vi "SwerveDriveSwerveWheel.vi"(0 "Wheel_Encoder":T1={"DevStatus"={"status"=FALSE, "code"=0, "source"=""}, "Analog Channel"=enum."Invalid"}, 1 "Wheel_Position":string="Numeric Array", 2 "Inputs":dbl[](array[numeric]), 3 "Length":dbl, 4 "Center":dbl, 5 "error in (no error)":errorcluster, 6 "Wheel_Offset":dbl, 7 "Width":dbl, 8 "MotorControlDevRef":T3={"DeviceStatus"={"status"=FALSE, "code"=0, "source"=""}, "Type"=enum."PWM", "PWM"={"PWM Channel"=enum."Invalid", "DeadBand"={"Name"="", "maxPositivePwm"=0, "minPositivePwm"=0, "centerPwm"=0, "maxNegativePwm"=0, "minNegativePwm"=0, "angularRange"=0}}, "CAN"={"Device Number"=0, "SetOutput VI Ref"=variant(refnum<vi> refnum), "GetOutput VI Ref"=variant(refnum<vi> refnum), "Enable VI Ref"=variant(refnum<vi> refnum), "Disable VI Ref"=variant(refnum<vi> refnum), "Data"=variant}, "Invert"=FALSE, "DIO PWM"={"PWM \"Enable\" Channel"=enum."Invalid", "DIOChannel"=enum."Invalid", "PWM Rate"=0.0}}) -> (19 "Speed":dbl)   [LabVIEW 2019, in "Swerve Drive.lvlib"]
uses:
  Swerve Drive.lvlib
  <vilib>/Rock Robotics/WPI/MotorControl/WPI_MotorControlDeviceRef.ctl
  <vilib>/Rock Robotics/WPI/MotorControl/WPI_MotorControlType.ctl
  <vilib>/Rock Robotics/SystemInterfaces/DIO/FPGA_DIOPWMChannel.ctl
  <vilib>/Rock Robotics/WPI/PWM/WPI_PWMDeadband.ctl
  <vilib>/Rock Robotics/SystemInterfaces/DIO/FPGA_DIOChannel.ctl
  <vilib>/Rock Robotics/WPI/AnalogChannel/WPI_AnalogChannelDevRef.ctl
  <vilib>/Rock Robotics/SystemInterfaces/AI/FPGA_AIChannel.ctl
  <vilib>/Rock Robotics/Network Tables/NT Write Number.vi
panel:
  out "error out":errorcluster
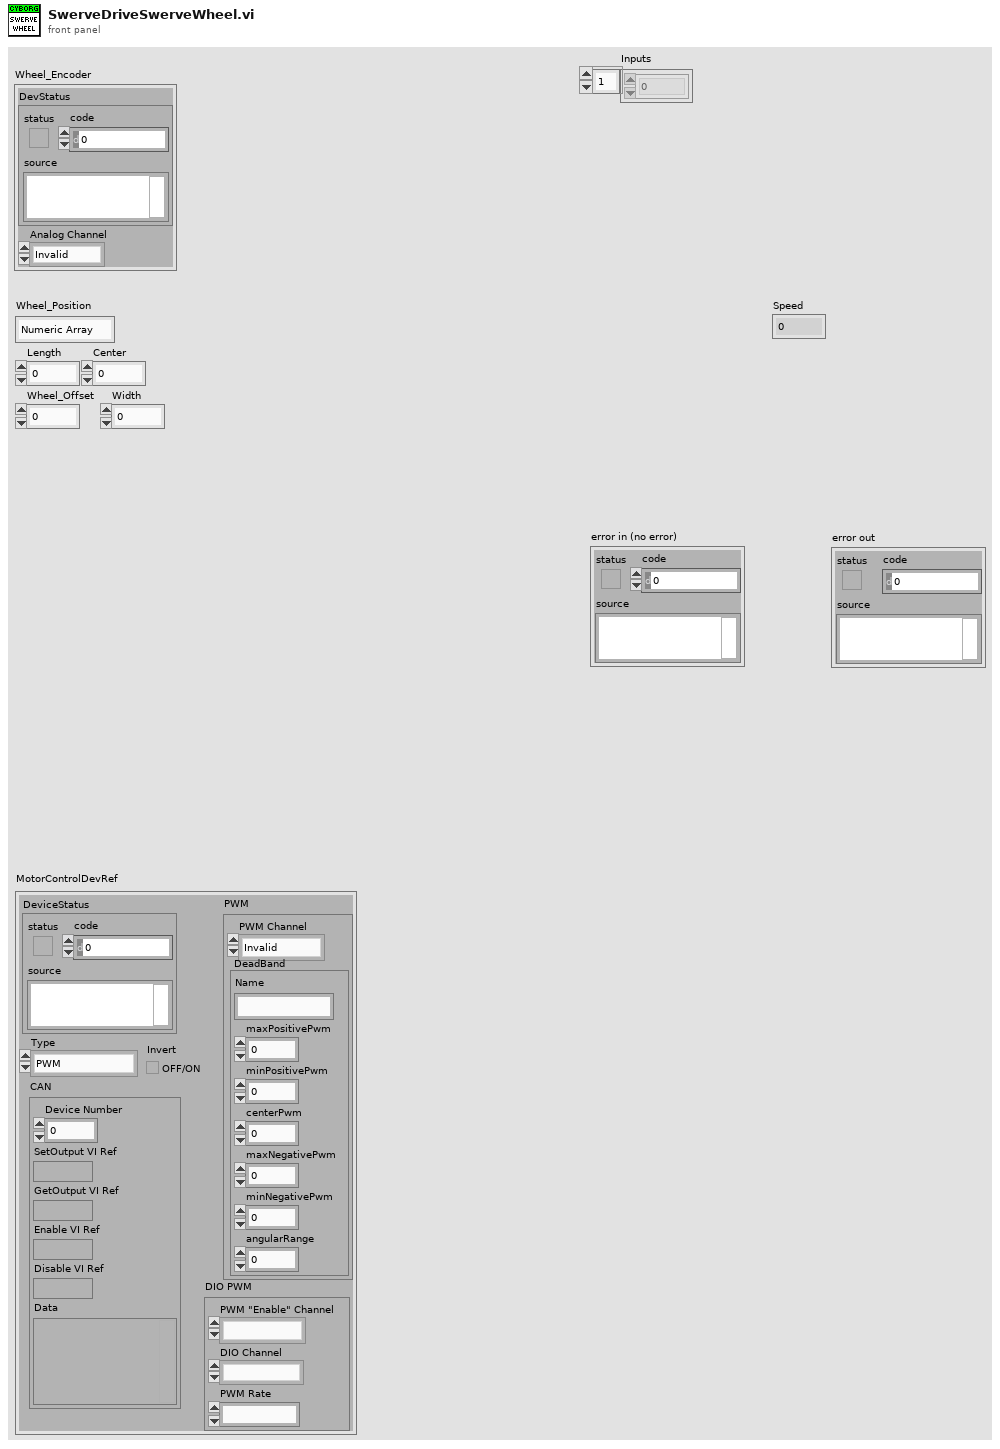
[diagram p1: front panel]
types:
  T1 = typedef "WPI_AnalogChannelDevRef.ctl" = cluster{"DevStatus":errorcluster, "Analog Channel":T2}
  T2 = typedef "FPGA_AIChannel.ctl" = enum8{"AI 0", "AI 1", "AI 2", "AI 3", "AI MXP 0", "AI MXP 1", "AI MXP 2", "AI MXP 3", "Invalid"}
  T3 = typedef "WPI_MotorControlDeviceRef.ctl" = cluster{"DeviceStatus":errorcluster, "Type":T4, "PWM":cluster{"PWM Channel":T5, "DeadBand":T6}, "CAN":cluster{"Device Number":u8, "SetOutput VI Ref":variant, "GetOutput VI Ref":variant, "Enable VI Ref":variant, "Disable VI Ref":variant, "Data":variant}, "Invert":bool, "DIO PWM":cluster{"PWM \"Enable\" Channel":T5, "DIOChannel":T7, "PWM Rate":dbl}}
  T4 = typedef "WPI_MotorControlType.ctl" = enum16{"PWM", "CAN", "DIO PWM"}
  T5 = typedef "FPGA_DIOPWMChannel.ctl" = enum8{"PWM 0", "PWM 1", "PWM 2", "PWM 3", "PWM 4", "PWM 5", "PWM 6", "PWM 7", "PWM 8", "PWM 9", "PWM MXP 0", "PWM MXP 1", "PWM MXP 2", "PWM MXP 3", "PWM MXP 4", "PWM MXP 5", "PWM MXP 6", "PWM MXP 7", "PWM MXP 8", "PWM MXP 9", "Invalid"}
  T6 = typedef "WPI_PWMDeadband.ctl" = cluster{"Name":string, "maxPositivePwm":i32, "minPositivePwm":i32, "centerPwm":i32, "maxNegativePwm":i32, "minNegativePwm":i32, "angularRange":u16}
  T7 = typedef "FPGA_DIOChannel.ctl" = enum8{"DIO 0", "DIO 1", "DIO 2", "DIO 3", "DIO 4", "DIO 5", "DIO 6", "DIO 7", "DIO 8", "DIO 9", "DIO MXP 0", "DIO MXP 1", "DIO MXP 2", "DIO MXP 3", "DIO MXP 4", "DIO MXP 5", "DIO MXP 6", "DIO MXP 7", "DIO MXP 8", "DIO MXP 9", "DIO MXP 10", "DIO MXP 11", "DIO MXP 12", "DIO MXP 13", "DIO MXP 14", "DIO MXP 15", "SPI Port CS1", "SPI Port CS2", "SPI Port CS3", "SPI Port MISO", "SPI Port MOSI", "Invalid"}
  T8 = enum16{"Z", "Y", "X", "Width/2", "Length/2", "Max"}
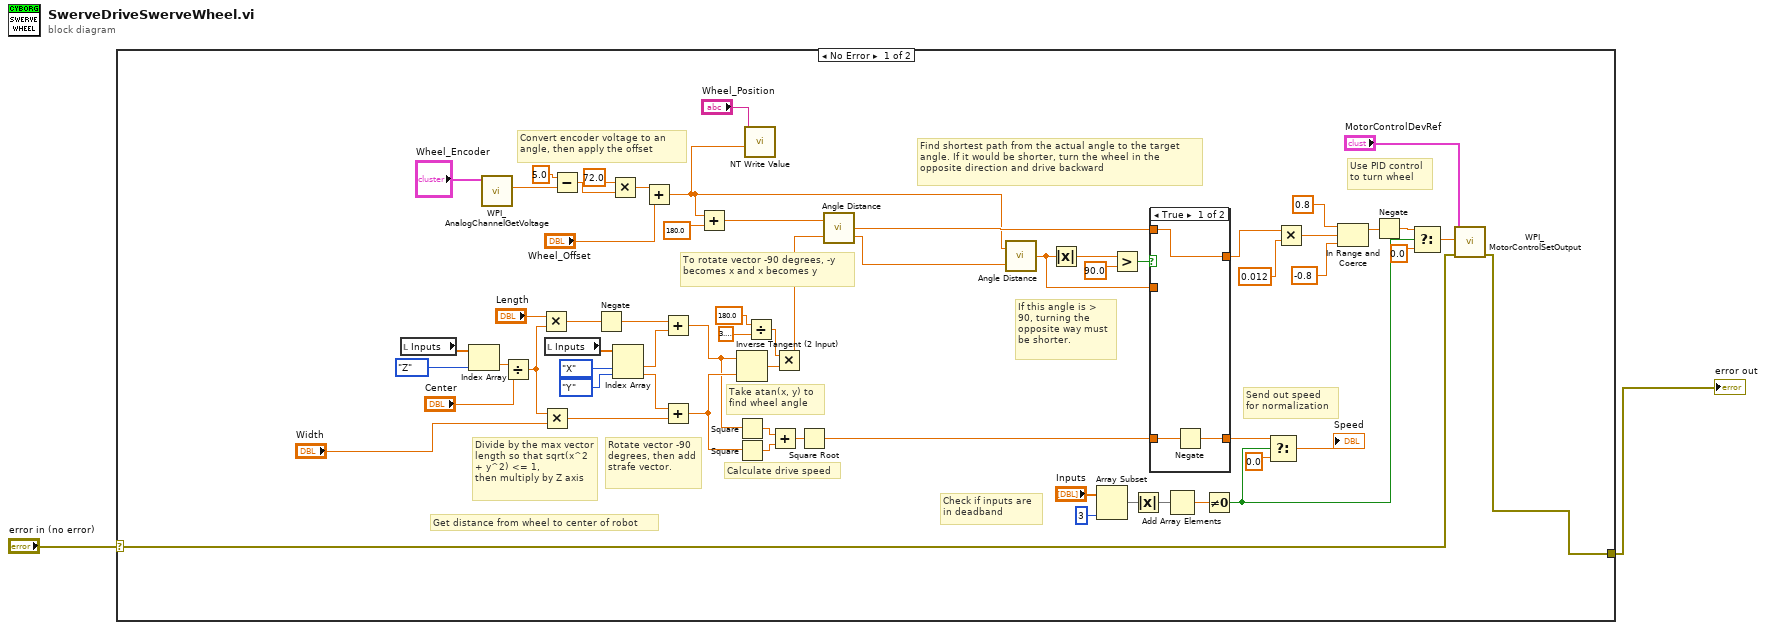
[diagram p0: block diagram]
diagram:
  n1 = case shown="No Error" "error in (no error)" {
    selector: "error in (no error)" -> [w11 w71]
    tunnel: [w65 w71] -> w1
    frame No Error {
      # "To rotate vector -90 degrees, -y becomes x and x becomes y"
      # "Divide by the max vector length so that sqrt(x^2 + y^2) <= 1,\nthen multiply by Z axis"
      # "Send out speed\nfor normalization"
      # "Check if inputs are\nin deadband"
      # "Convert encoder voltage to an angle, then apply the offset"
      # "If this angle is > 90, turning the opposite way must be shorter."
      # "Use PID control\nto turn wheel"
      # "Find shortest path from the actual angle to the target angle. If it would be shorter, turn the wheel in the opposite direction and drive backward"
      # "Take atan(x, y) to find wheel angle"
      # "Calculate drive speed"
      # "Rotate vector -90 degrees, then add strafe vector."
      # "Get distance from wheel to center of robot"
      n2 = local read "Inputs"() -> (w39:dbl[])
      n3 = Index Array(array=w39, index=T8."Z") -> (element=w38:dbl)
      n4 = call <vilib>:"WPI_AnalogChannelGetVoltage.vi"("AIDeviceRef"="Wheel_Encoder") -> ("Voltage"=w25:dbl)  [unwired: 8 in, 2 out]
      n5 = Divide(x=w38, y="Center") -> (x/y=w37:dbl)
      n6 = Multiply(x="Length", y=w37) -> (x*y=w28:dbl)
      n7 = Multiply(x=w37, y="Width") -> (x*y=w34:dbl)
      n8 = local read "Inputs"() -> (w36:dbl[])
      n9 = Subtract(x=5.0, y=w25) -> (x-y=w19:dbl)
      n10 = Negate(x=w28) -> (-x=w27:dbl)
      n11 = Multiply(x=72.0 ("y"), y=w19) -> (x*y=w50:dbl)
      n12 = Index Array(array=w36, index #1=T8."X", index #2=T8."Y") -> (element #1=w32:dbl, element #2=w33:dbl)
      n13 = Add(x=w50, y="Wheel_Offset") -> (x+y=w12:dbl)
      n14 = Add(x=w27, y=w32) -> (x+y=w30:dbl)
      n15 = Add(x=w33, y=w34) -> (x+y=w31:dbl)
      n16 = Add(x=w12, y=180.0 ("f")) -> (x+y=w47:dbl)
      n17 = Inverse Tangent (2 Input)(1:w31, 2:w30) -> (0:w61:dbl)
      n18 = Square(x=w30) -> (x^2=w35:dbl)
      n19 = Square(x=w31) -> (x^2=w60:dbl)
      n20 = call-poly <vilib>:"NT Write Value.vi"("Numeric"=w12, "Name"="Wheel_Position") -> ()  [unwired: 9 in, 1 out]
      n21 = Divide(x=180.0 ("y"), y=3.141592653589793) -> (x/y=w58:dbl)
      n22 = Add(x=w35, y=w60) -> (x+y=w59:dbl)
      n23 = Multiply(x=w58, y=w61) -> (x*y=w29:dbl)
      n24 = Square Root(x=w59) -> (sqrt(x)=w52:dbl)
      n25 = call "Angle Distance.vi"("target angle"=w29, "current angle"=w47) -> ("distance"=w20:dbl)
      n26 = call "Angle Distance.vi"("target angle"=w29, "current angle"=w12) -> ("distance"=w53:dbl)
      n27 = Absolute Value(x=w53) -> (abs(x)=w54:dbl)
      n28 = Array Subset(array="Inputs", length=3) -> (w46:dbl[])  [unwired: 1 in]
      n29 = Greater?(x=w54, y=90.0) -> (0:w43:bool)
      n30 = Absolute Value(x=w46) -> (abs(x)=w40:dbl[])
      n31 = case shown="True" w43 {
        tunnel: w20 -> [w66 _]
        tunnel: w53 -> [_ w70]
        tunnel: [w67 w69] -> w45
        tunnel: w52 -> [w68 w69]
        tunnel: [w66 w70] -> w14
        frame True {
          n32 = Negate(x=w68) -> (-x=w67:dbl)
        }
        frame False {
        }
      }
      n33 = Add Array Elements(numeric array=w40) -> (sum=w62:dbl)
      n34 = Not Equal To 0?(x=w62) -> (x != 0?=w42:bool)
      n35 = Select(t=w45, s=w42, f=0.0) -> (s? t:f=→"Speed":dbl)
      n36 = Multiply(x=w14, y=0.012) -> (x*y=w17:dbl)
      n37 = In Range and Coerce(upper limit=0.8, x=w17, lower limit=-0.8) -> (coerced(x)=w18:dbl)  [unwired: 1 out]
      n38 = Negate(x=w18) -> (-x=w41:dbl)
      n39 = Select(t=w41, s=w42, f=0.0) -> (s? t:f=w49:dbl)
      n40 = call <vilib>:"WPI_MotorControlSetOutput.vi"("error in (no error)"=w11, "Output"=w49, "MotorControlDevRef"="MotorControlDevRef") -> ("error out"=w65:errorcluster)  [unwired: 6 in, 2 out]
    }
    frame Error {
    }
  }
  "error out" <- w1
